vi "Main_Module.vi"(0 "File_hierarchy":string(tree)) -> ()   [LabVIEW 2023]
doc: "This is the main vi that performs based calci operation"
uses:
  Controls/Queue_Operation_Select.ctl
  Controls/State_and_Data.ctl
  Controls/Culci_Data.ctl
  Controls/Notifier_Operation_Select.ctl
panel:
  out "Error_Out":errorcluster
  in  "Error_In":errorcluster
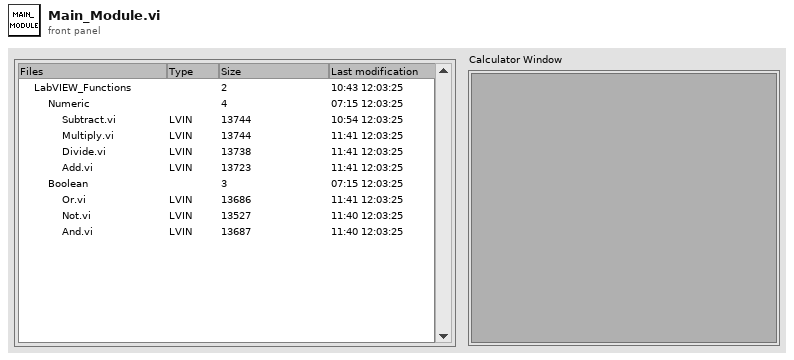
[diagram p1: front panel]
types:
  T1 = typedef "Notifier_Operation_Select.ctl" = enum16{"Obtain_Notifier", "Send_Notification", "Get_Notification_Status", "Release_Notifier"}
  T2 = typedef "Queue_Operation_Select.ctl" = enum16{"Obtain_Queue", "Enqueue", "Enqueue_First", "Enqueue_N", "Lossy_Enqueue", "Preview", "Queue_Status", "Dequeue", "Flush", "Release_Queue"}
  T3 = typedef "Culci_Data.ctl" = cluster{"File_hierarchy_Reference":refnum<vi>, "Tag":string, "State_and_Data":T4}
  T4 = typedef "State_and_Data.ctl" = cluster{"State":string, "Data":variant}
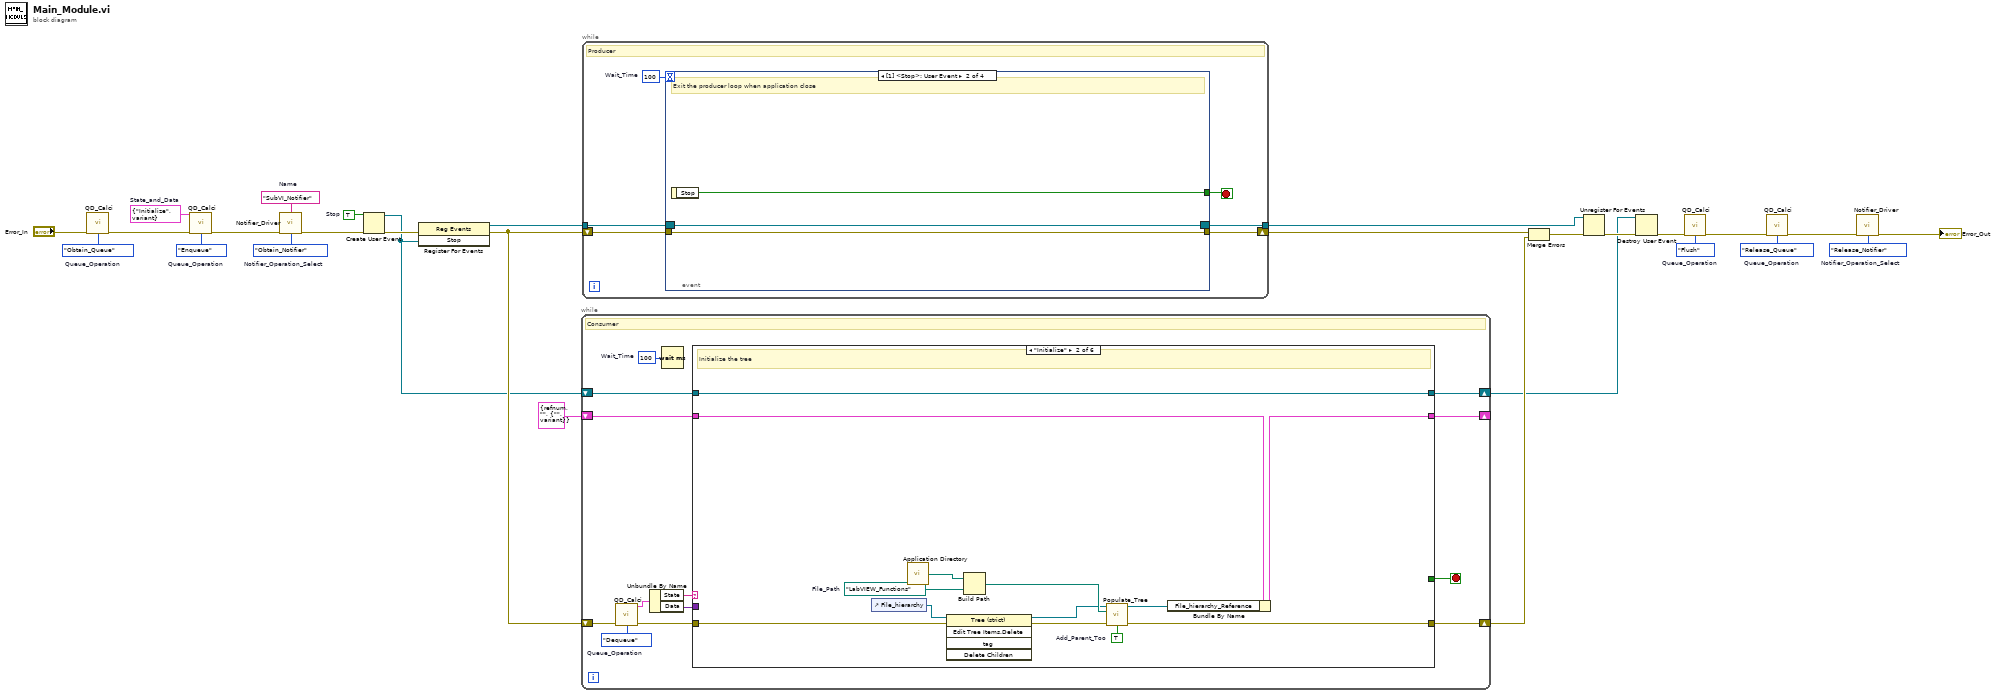
[diagram p0: block diagram]
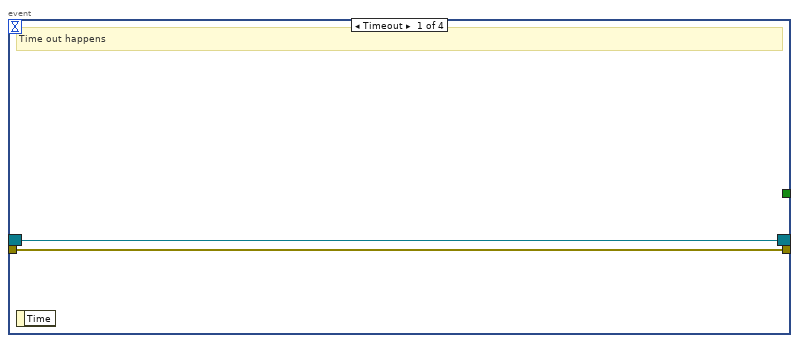
[diagram p2: hidden frame]
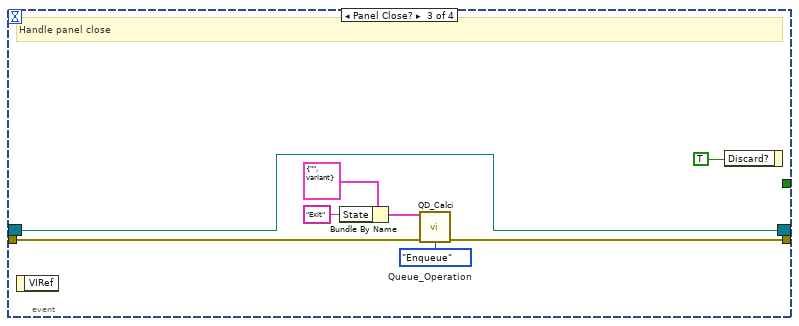
[diagram p3: hidden frame]
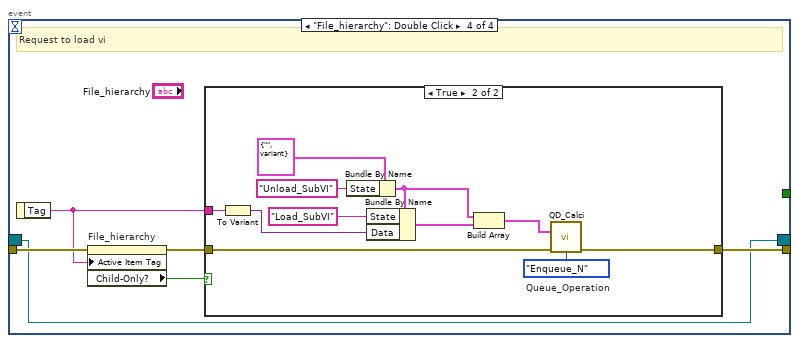
[diagram p4: hidden frame]
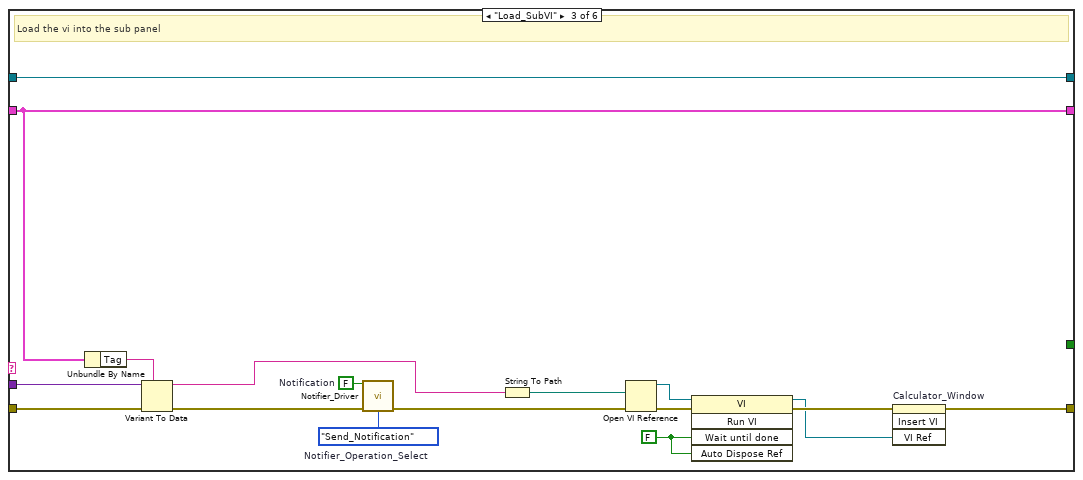
[diagram p7: hidden frame]
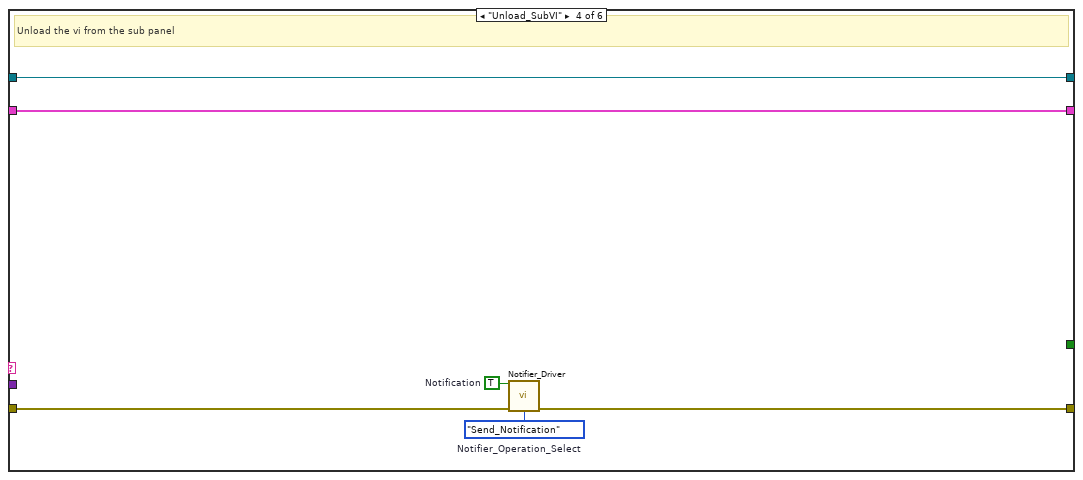
[diagram p8: hidden frame]
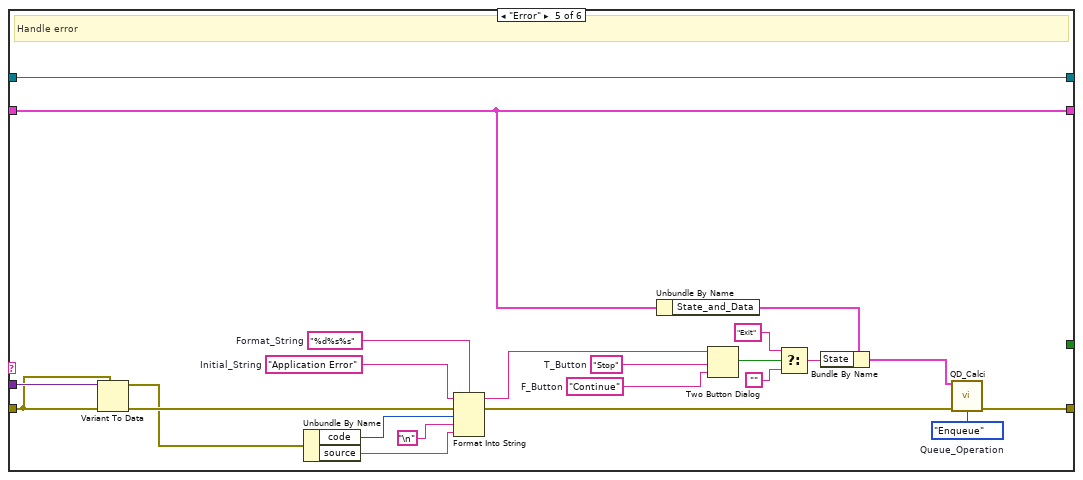
[diagram p9: hidden frame]
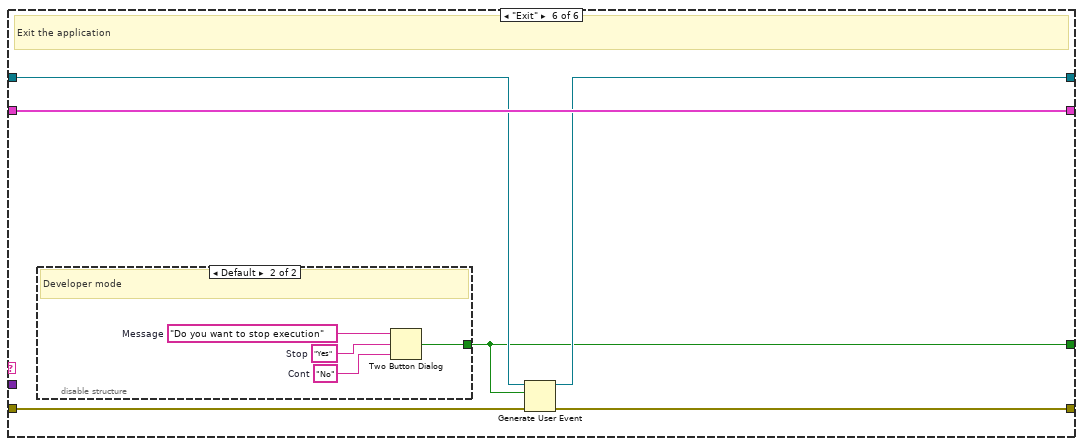
[diagram p10: hidden frame]
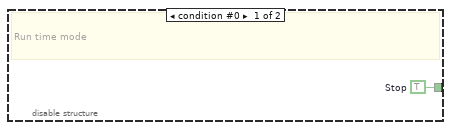
[diagram p11: hidden frame]
diagram:
  w1 = Notifier_Operation_Select."Release_Notifier"  # Notifier_Operation_Select
  w3 = Queue_Operation_Select."Release_Queue"  # Queue_Operation
  w5 = Queue_Operation_Select."Flush"  # Queue_Operation
  w17 = TRUE  # Stop
  w19 = "SubVI_Notifier"  # Name
  w20 = Notifier_Operation_Select."Obtain_Notifier"  # Notifier_Operation_Select
  w24 = T4 {"State"="Initialize", "Data"=variant}  # State_and_Data
  w25 = Queue_Operation_Select."Enqueue"  # Queue_Operation
  w26 = Queue_Operation_Select."Obtain_Queue"  # Queue_Operation
  n1 = call "QD_Calci.vi"("Error_In"="Error_In", "Queue_Operation"=w26) -> ("Error_Out"=w27:errorcluster)  [unwired: 11 in, 2 out]
  n2 = call "QD_Calci.vi"("State_and_Data_In"=w24, "Error_In"=w27, "Queue_Operation"=w25) -> ("Error_Out"=w23:errorcluster)  [unwired: 10 in, 2 out]
  n3 = call "Notifier_Driver.vi"("Name"=w19, "Error_In"=w23, "Notifier_Operation_Select"=w20) -> ("Error_Out"=w21:errorcluster)  [unwired: 11 in, 1 out]
  n4 = Create User Event(user event datatype=w17, error in=w21) -> (user event=w9:refnum<user-event>, error out=w18:errorcluster)
  n5 = register-events(error in=w18, w9) -> (reference out=w15:refnum<event-registration>, error out=w16:errorcluster)  [unwired: 1 in]
  n6 = while {
    shift-right: [w33] -> w8
    shift-left: w9 -> [w34]
    shift-right: [w32] -> _
    shift-left: T3 {"File_hierarchy_Reference"=refnum, "Tag"="", "State_and_Data"={"State"="", "Data"=variant}} -> [w35]
    shift-right: [w31] -> w13
    shift-left: w16 -> [w41]
    stop <- w30 stop-if-true
    w29 = u32 100  # Wait_Time
    w39 = Queue_Operation_Select."Dequeue"  # Queue_Operation
    # "Consumer"
    n7 = call "QD_Calci.vi"("Error_In"=w41, "Queue_Operation"=w39) -> ("State_and_Data_Out"=w38:T4, "Error_Out"=w40:errorcluster)  [unwired: 11 in, 1 out]
    n8 = Unbundle By Name(w38) -> ("State"=w37:string, "Data"=w36:variant)
    n9 = Wait (ms)(milliseconds to wait=w29) -> ()  [unwired: 1 out]
    n10 = case shown="\"Initialize\"" w37 {
      tunnel: [w44 w57 w72 w79 w84 w107] -> w31
      tunnel: w40 -> [w44 w56 w74 w80 w101 w109]
      tunnel: w36 -> [_ _ w73 _ w102 _]
      tunnel: w35 -> [w43 w50 w59 w75 w86 w108]
      tunnel: [w43 w49 w59 w75 w86 w108] -> w32
      tunnel: w34 -> [w42 w47 w70 w77 w103 w106]
      tunnel: [w42 w47 w70 w77 w103 w105] -> w33
      tunnel: [_ _ _ _ _ w104] -> w30
      frame Default {
      }
      frame "Initialize" {
        w45 = TRUE  # Add_Parent_Too
        w53 = path "LabVIEW_Functions"  # File_Path
        # "Initialize the tree"
        n11 = control-ref of="File_hierarchy"() -> (w46:refnum<vi>)
        n12 = call <vilib>:"Application Directory.vi"() -> ("Application Directory"=w54:path)
        n13 = invoke class="Tree (strict)" method="Edit Tree Items.Delete"(reference=w46, error in=w56) -> (reference out=w51:refnum<vi>, error out=w52:errorcluster)  [unwired: 3 in, 3 out]
        n14 = Build Path(base path=w54, name or relative path=w53) -> (appended path=w55:path)
        n15 = call "Populate_Tree.vi"("Reference_In"=w51, "File_Path"=w55, "Error_In"=w52, "Add_Parent_Too"=w45) -> ("Reference_Out"=w48:refnum<vi>, "Error_Out"=w57:errorcluster)  [unwired: 10 in]
        n16 = Bundle By Name(cluster=w50, "File_hierarchy_Reference"=w48) -> (w49:T3)
      }
      frame "Load_SubVI" {
        w60 = FALSE ("Wait Until Done")
        w67 = FALSE  # Notification
        w68 = Notifier_Operation_Select."Send_Notification"  # Notifier_Operation_Select
        # "Load the vi into the sub panel"
        n17 = Unbundle By Name(w59) -> ("Tag"=w71:string)
        n18 = Variant To Data(error in=w74, type=w71, Variant=w73) -> (data=w66:string, error out=w69:errorcluster)
        n19 = call "Notifier_Driver.vi"("Notification"=w67, "Error_In"=w69, "Notifier_Operation_Select"=w68) -> ("Error_Out"=w58:errorcluster)  [unwired: 11 in, 1 out]
        n20 = String To Path(string=w66) -> (path=w61:path)
        n21 = Open VI Reference(vi path=w61, error in (no error)=w58) -> (vi reference=w63:refnum<vi>, error out=w65:errorcluster)  [unwired: 4 in]
        n22 = invoke class="VI" method="Run VI"(reference=w63, error in=w65, "Wait until done"=w60, "Auto Dispose Ref"=w60) -> (reference out=w62:refnum<vi>, error out=w64:errorcluster)  [unwired: 1 in, 3 out]
        n23 = invoke on="Calculator_Window" class="SubPnl" method="Insert VI"(error in=w64, "VI Ref"=w62) -> (error out=w72:errorcluster)  [unwired: 2 in, 3 out]
      }
      frame "Unload_SubVI" {
        w76 = TRUE  # Notification
        w78 = Notifier_Operation_Select."Send_Notification"  # Notifier_Operation_Select
        # "Unload the vi from the sub panel"
        n24 = call "Notifier_Driver.vi"("Notification"=w76, "Error_In"=w80, "Notifier_Operation_Select"=w78) -> ("Error_Out"=w79:errorcluster)  [unwired: 11 in, 1 out]
      }
      frame "Error" {
        w83 = Queue_Operation_Select."Enqueue"  # Queue_Operation
        w96 = "%d%s%s"  # Format_String
        w97 = "Application Error"  # Initial_String
        w98 = "Stop"  # T_Button
        w99 = "Continue"  # F_Button
        # "Handle error"
        n25 = Variant To Data(error in=w101, type=w101, Variant=w102) -> (data=w82:errorcluster, error out=w88:errorcluster)
        n26 = Unbundle By Name(w82) -> ("code"=w94:i32, "source"=w93:string)
        n27 = Format Into String(format string=w96, initial string=w97, error in=w88, w94, "\n", w93) -> (resulting string=w100:string, error out=w87:errorcluster)
        n28 = Unbundle By Name(w86) -> ("State_and_Data"=w85:T4)
        n29 = Two Button Dialog(message=w100, 1:w99, 2:w98) -> (T button?=w91:bool)
        n30 = Select(t="Exit" ("State"), s=w91, f="") -> (s? t:f=w89:string)
        n31 = Bundle By Name(cluster=w85, "State"=w89) -> (w81:T4)
        n32 = call "QD_Calci.vi"("State_and_Data_In"=w81, "Error_In"=w87, "Queue_Operation"=w83) -> ("Error_Out"=w84:errorcluster)  [unwired: 10 in, 2 out]
      }
      frame "Exit" {
        # "Exit the application"
        n33 = disable-structure shown="Default" {
          disable-tunnel: [w110 w114] -> w104
          frame condition #0 {
            w110 = TRUE  # Stop
            # "Run time mode"
          }
          frame condition #1 (active) {
            w111 = "No"  # Cont
            w112 = "Yes"  # Stop
            w113 = "Do you want to stop execution"  # Message
            # "Developer mode"
            n34 = Two Button Dialog(message=w113, 1:w111, 2:w112) -> (T button?=w114:bool)
          }
        }
        n35 = Generate User Event(user event=w106, event data cluster=w104, error in=w109) -> (user event out=w105:refnum<user-event>, error out=w107:errorcluster)  [unwired: 1 in]
      }
    }
  }
  n36 = while {
    tunnel: w15 -> [w119]
    shift-right: [w117] -> w14
    shift-left: w16 -> [w120]
    tunnel: [w115] -> w11
    stop <- w118 stop-if-true
    w116 = 100  # Wait_Time
    # "Producer"
    n37 = event shown="[1] <Stop>: User Event" {
      selector: w119 -> [w121 w123 w126 w134]
      dyn-events: [w121 w123 w126 w134] -> w115
      timeout: w116 -> [_ _ _ _]
      tunnel: w120 -> [w122 w125 w130 w138]
      tunnel: [w122 w125 w129 w139] -> w117
      tunnel: [_ w124 _ _] -> w118
      event Timeout {
        # "Time out happens"
        n38 = event-data() -> ()  [unwired: 1 in, 1 out]
      }
      event User Event {
        # "Exit the producer loop when application close"
        n39 = event-data() -> ("Stop"=w124:bool)  [unwired: 1 in]
      }
      event Panel Close? {
        w131 = Queue_Operation_Select."Enqueue"  # Queue_Operation
        # "Handle panel close"
        n40 = event-data() -> ()  [unwired: 1 in, 1 out]
        n41 = Bundle By Name(cluster=T4 {"State"="", "Data"=variant} ("State_and_Data"), "State"="Exit") -> (w128:T4)
        n42 = call "QD_Calci.vi"("State_and_Data_In"=w128, "Error_In"=w130, "Queue_Operation"=w131) -> ("Error_Out"=w129:errorcluster)  [unwired: 10 in, 2 out]
        n43 = event-data("Discard?"=TRUE) -> ()  [unwired: 1 in, 1 out]
      }
      event "File_hierarchy": Double Click {
        # "Request to load vi"
        n44 = event-data() -> ("Tag"=w136:string)  [unwired: 1 in]
        n45 = property on="File_hierarchy" class="Tree (strict)"(error in=w138, "Active Item Tag"=w136) -> (error out=w137:errorcluster, "Child-Only?"=w135:bool)  [unwired: 1 in, 1 out]
        n46 = case shown="True" w135 {
          tunnel: [w140 w151] -> w139
          tunnel: w137 -> [w140 w142]
          tunnel: w136 -> [_ w141]
          frame False {
          }
          frame True {
            w148 = Queue_Operation_Select."Enqueue_N"  # Queue_Operation
            n47 = To Variant(anything=w141) -> (Variant=w149:variant)
            n48 = Bundle By Name(cluster=T4 {"State"="", "Data"=variant} ("State_and_Data"), "State"="Unload_SubVI") -> (w144:T4)
            n49 = Bundle By Name(cluster=w144, "State"="Load_SubVI", "Data"=w149) -> (w145:T4)
            n50 = Build Array(w144, w145) -> (w143:T4[])
            n51 = call "QD_Calci.vi"("State_and_Data_N_In"=w143, "Error_In"=w142, "Queue_Operation"=w148) -> ("Error_Out"=w151:errorcluster)  [unwired: 10 in, 2 out]
          }
        }
      }
    }
  }
  n52 = Merge Errors(w14, w13) -> (w12:errorcluster)
  n53 = Unregister For Events(event registration refnum=w11, error in=w12) -> (error out=w10:errorcluster)
  n54 = Destroy User Event(user event=w8, error in=w10) -> (error out=w7:errorcluster)
  n55 = call "QD_Calci.vi"("Error_In"=w7, "Queue_Operation"=w5) -> ("Error_Out"=w6:errorcluster)  [unwired: 11 in, 2 out]
  n56 = call "QD_Calci.vi"("Error_In"=w6, "Queue_Operation"=w3) -> ("Error_Out"=w4:errorcluster)  [unwired: 11 in, 2 out]
  n57 = call "Notifier_Driver.vi"("Error_In"=w4, "Notifier_Operation_Select"=w1) -> ("Error_Out"=→"Error_Out":errorcluster)  [unwired: 12 in, 1 out]
